vi "_Pop Up.vi"() -> (2 "Msg Strategy":refnum<class "Msg Strategy.lvclass">)   [LabVIEW 2021, in "jettl Msg Pop Up.lvlib"]
uses:
  jettl Msg Pop Up.lvlib
  jettl/Msg Strategy/Msg Strategy.lvclass
  Pop Up Msg Strategy/Pop Up Msg Strategy.lvclass
  C:/git/jettl/src/Hello World/jettl Msg Pop Up/Pop Up Msg Strategy/Pop Up Msg Strategy.lvclass
  C:/git/jettl/src/jettl/Msg Strategy/Msg Strategy.lvclass
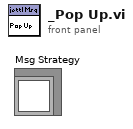
[diagram p1: front panel]
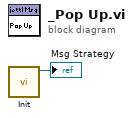
[diagram p0: block diagram]
diagram:
  n1 = call "Init.vi"() -> ("Pop Up Msg Strategy out"=→"Msg Strategy":refnum<class "Pop Up Msg Strategy.lvclass">)  [unwired: 11 in]
